vi "CreateXML.vi"(6 "Standalone? (T)":bool caption="独立？(T)", 8 "error in (no error)":errorcluster caption="错误输入（无错误）", 10 "XML Input":string caption="XML输入", 11 "XML File Path":path caption="XML文件路径") -> (0 "error out":errorcluster caption="错误输出", 2 "XML String":string caption="XML字符串", 3 "XML File Path(duplicate)":path caption="XML文件路径（副本）")   [LabVIEW 2018]
panel:
  in  "Prompt":string="选择XML文件路径" caption="提示"
  out "连接的字符串":string
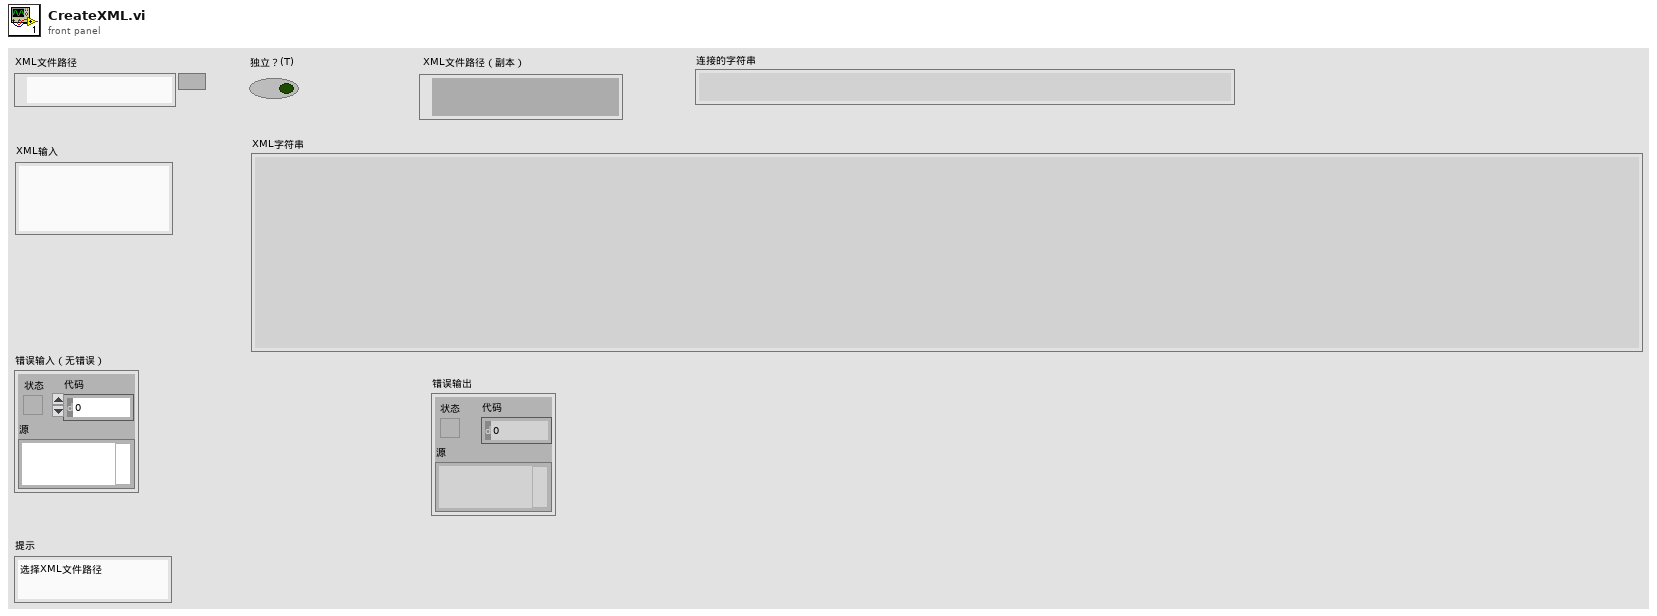
[diagram p1: front panel]
types:
  T1 = enum16{"open", "open or create", "create or replace", "create", "open (read only)"}
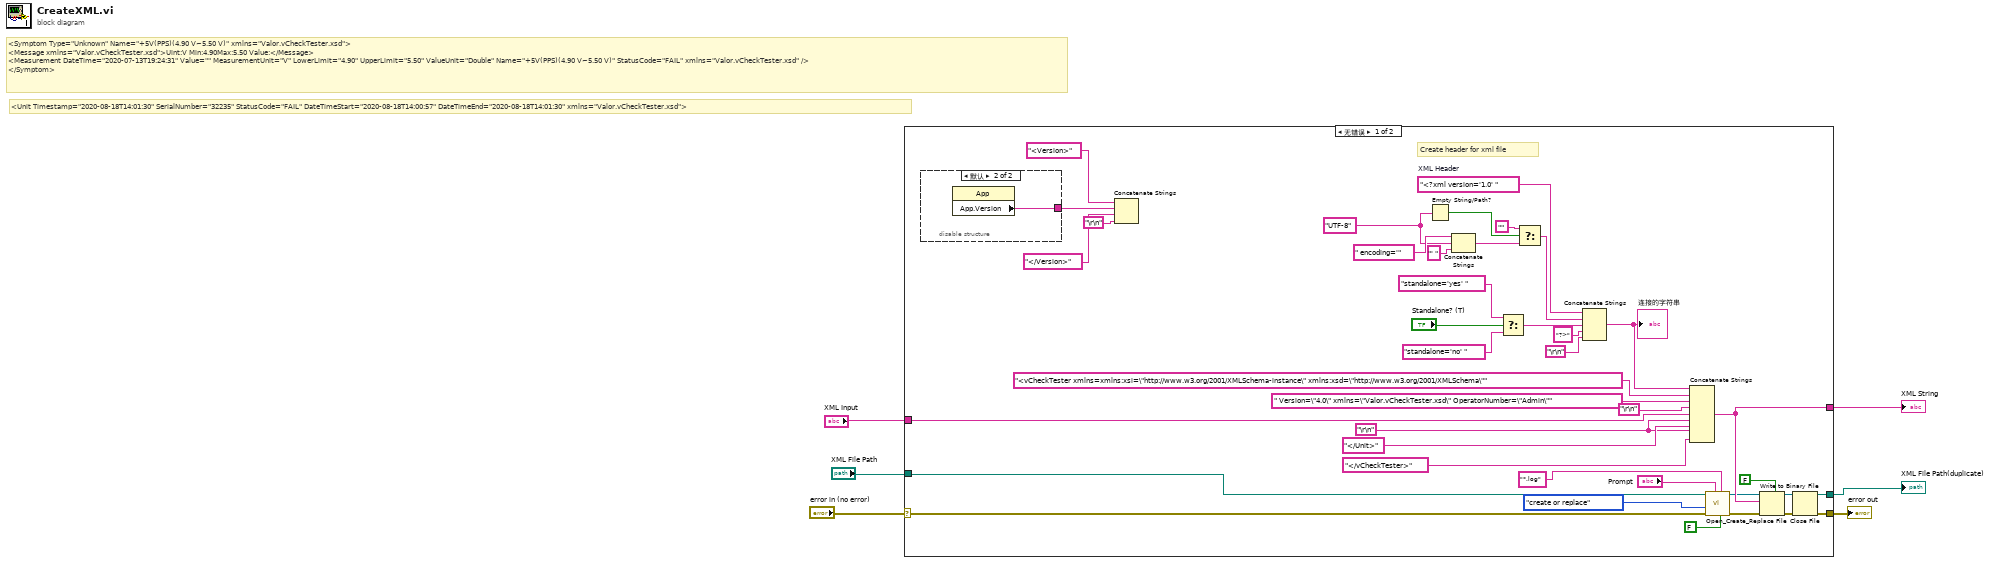
[diagram p0: block diagram]
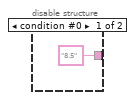
[diagram p2: hidden frame]
diagram:
  # "<Symptom Type=\"Unknown\" Name=\"+5V(PPS)(4.90 V~5.50 V)\" xmlns=\"Valor.vCheckTester.xsd\">\n<Message xmlns=\"Valor.vCheckTester.xsd\">Uint:V Min:4.90Max:5.50 Value:</Message>\n<Measurement DateTime=\"2020-07-13T19:24:31\" Value=\"\" MeasurementUnit=\"V\" LowerLimit=\"4.90\" UpperLimit=\"5.50\" ValueUnit=\"Double\" Name=\"+5V(PPS)(4.90 V~5.50 V)\" StatusCode=\"FAIL\" xmlns=\"Valor.vCheckTester.xsd\" />\n</Symptom>"
  # "<Unit Timestamp=\"2020-08-18T14:01:30\" SerialNumber=\"32235\" StatusCode=\"FAIL\" DateTimeStart=\"2020-08-18T14:00:57\" DateTimeEnd=\"2020-08-18T14:01:30\" xmlns=\"Valor.vCheckTester.xsd\">"
  n1 = case shown="无错误" "error in (no error)" {
    selector: "error in (no error)" -> [w20 w51]
    tunnel: [w21 w51] -> w4
    tunnel: "XML Input" -> [w31 w50]
    tunnel: [w19 w50] -> w3
    tunnel: [w15 w49] -> w2
    tunnel: "XML File Path" -> [w25 w49]
    frame No Error {
      w39 = "UTF-8" ("XML Encoding")
      w8 = "\r\n"
      w46 = "<?xml version='1.0' "  # XML Header
      # "Create header for xml file"
      n2 = disable-structure shown="默认" {
        disable-tunnel: ["8.5" ("App.Version") w48] -> w29
        frame condition #0 {
        }
        frame condition #1 (active) {
          n3 = property class="App"() -> ("App.Version"=w48:string)  [unwired: 2 in, 2 out]
        }
      }
      n4 = Concatenate Strings("<Version>", w29, "</Version>", "\r\n") -> ()  [unwired: 1 out]
      n5 = Empty String/Path?(string/path=w39) -> (empty?=w38:bool)
      n6 = Concatenate Strings(" encoding='", w39, "' " ("Substring")) -> (w37:string)
      n7 = Select(t="standalone='yes' " ("Substring"), s="Standalone? (T)", f="standalone='no' " ("Substring")) -> (s? t:f=w32:string)
      n8 = Select(t="", s=w38, f=w37) -> (s? t:f=w35:string)
      n9 = Concatenate Strings(w46, w35, w32, "?>" ("Substring"), "\r\n") -> (w43:string)
      "连接的字符串" <- w43
      n10 = Concatenate Strings(w43, "<vCheckTester xmlns=xmlns:xsi=\"http://www.w3.org/2001/XMLSchema-instance\" xmlns:xsd=\"http://www.w3.org/2001/XMLSchema\"" ("Substring"), " Version=\"4.0\" xmlns=\"Valor.vCheckTester.xsd\" OperatorNumber=\"Admin\"" ("字符串"), "\r\n", w31, w8, "</Unit>", w8, "</vCheckTester>") -> (w19:string)
      n11 = call <vilib>:"Open_Create_Replace File.vi"("advisory dialog? (display:T)"=FALSE, "pattern"="*.log", "prompt"="Prompt", "error in (no error)"=w20, "function (open:0)"=T1."create or replace", "file path"=w25) -> ("error out"=w23:errorcluster, "refnum"=w18:refnum<file>)  [unwired: 2 in, 2 out]
      n12 = Write to Binary File(file (use dialog)=w18, data=w19, error in=w23, 5:FALSE ("prepend array or string size? (T)")) -> (refnum out=w16:refnum<file>, error out=w22:errorcluster)  [unwired: 3 out]
      n13 = Close File(refnum=w16, error in=w22) -> (path=w15:path, error out=w21:errorcluster)
    }
    frame Error {
    }
  }
  "error out" <- w4
  "XML String" <- w3
  "XML File Path(duplicate)" <- w2
